vi "Get SGL.vi"(8 "error in (no error)":errorcluster, 9 "Data Type (default value)":sgl=nan, 10 "Offset":i32, 11 "JSON":string) -> (0 "error out":errorcluster, 1 "Number":sgl format="%.2f", 2 "Offset past match":i32)   [LabVIEW 2024, in "JSONtext.lvlib"]
uses:
  JSONtext.lvlib
  String Subset.vi
  Advance past Number.vi
  Parsing Error in converting to LabVIEW type.vi
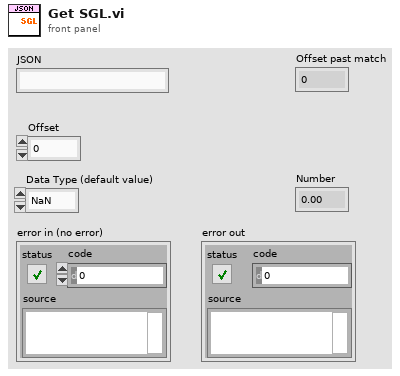
[diagram p1: front panel]
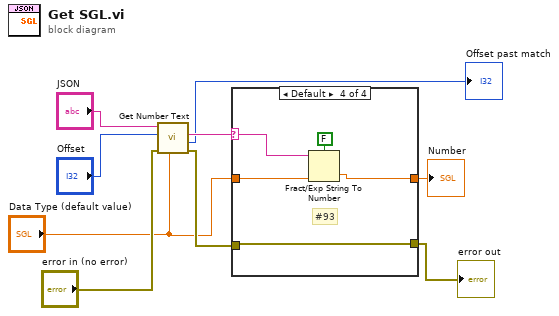
[diagram p0: block diagram]
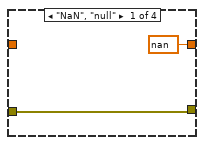
[diagram p2: hidden frame]
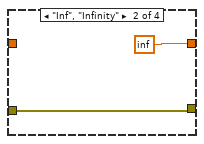
[diagram p3: hidden frame]
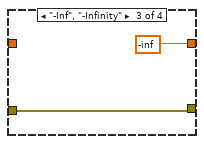
[diagram p4: hidden frame]
diagram:
  n1 = call "Get Number Text.vi"("LV Type"="Data Type (default value)", "error in (no error)"="error in (no error)", "Offset"="Offset", "JSON"="JSON") -> ("error out"=w6:errorcluster, "Offset past match"=→"Offset past match":i32, "Number Text"=w4:string)  [unwired: 4 in, 1 out]
  n2 = case shown="Default" w4 {
    selector: w4 -> [_ _ _ w16]
    tunnel: [sgl nan ("default value 1") sgl inf ("default value 1") sgl -inf ("default value 1") w18] -> w3
    tunnel: w6 -> [w11 w12 w14 w17]
    tunnel: [w11 w12 w14 w17] -> w5
    tunnel: "Data Type (default value)" -> [_ _ _ w19]
    frame "NaN", "null" {
    }
    frame "Inf", "Infinity" {
    }
    frame "-Inf", "-Infinity" {
    }
    frame Default {
      # "#93"
      n3 = Fract/Exp String To Number(use system decimal point (T)=FALSE, string=w16, default (0 dbl)=w19) -> (number=w18:sgl)  [unwired: 1 in, 1 out]
    }
  }
  "error out" <- w5
  "Number" <- w3
